vi "Boolean.vi"() -> ()   [LabVIEW 2020]
panel:
  out "0, 1":i16
  out "logical OR":bool
  out "logical AND":bool
  out "result":bool
  out ".not. (x .or. y)?":bool
  out "x .xor. y?":bool
  out "x .or. y?":bool
  out ".not. (x .and. y)?":bool
  out ".not. x?":bool
  in  "Boolean":bool
  out "x .and. y?":bool
  in  "x":bool
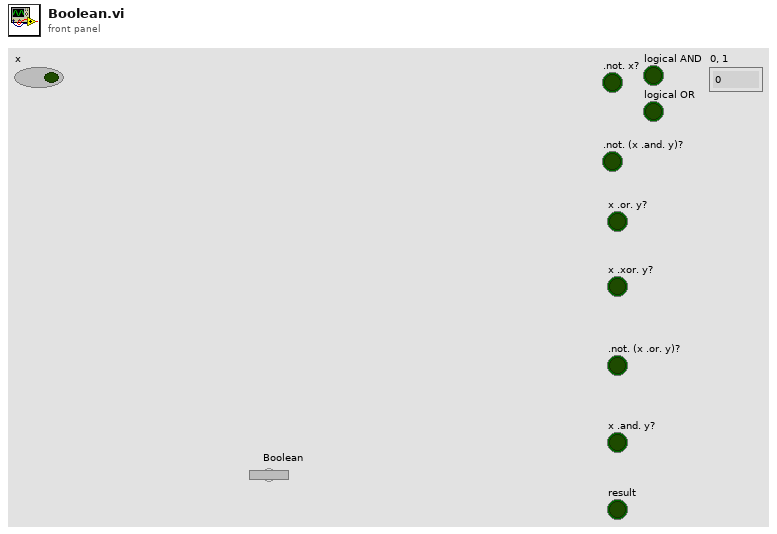
[diagram p1: front panel]
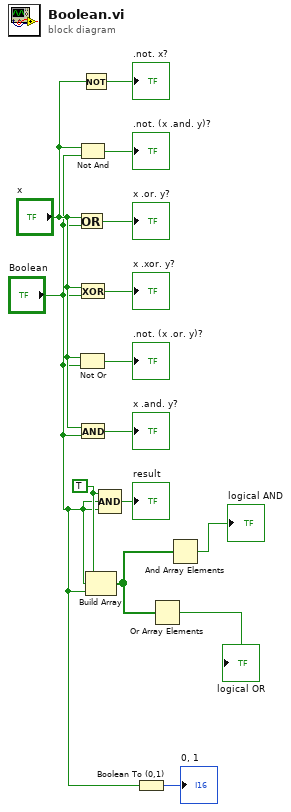
[diagram p0: block diagram]
diagram:
  w6 = TRUE
  n1 = Or(x="x", y="Boolean") -> (x .or. y?=→"x .or. y?":bool)
  n2 = Not Or(1:"Boolean", 2:"x") -> (0:→".not. (x .or. y)?":bool)
  n3 = Not And(1:"Boolean", 2:"x") -> (0:→".not. (x .and. y)?":bool)
  n4 = Exclusive Or(1:"Boolean", 2:"x") -> (0:→"x .xor. y?":bool)
  n5 = And(x="x", y="Boolean") -> (x .and. y?=→"x .and. y?":bool)
  n6 = Not(x="x") -> (.not. x?=→".not. x?":bool)
  n7 = Build Array(w6, "Boolean", "Boolean") -> (w5:bool[])
  n8 = Compound Arithmetic op=AND(w6, "Boolean", "Boolean") -> (→"result":bool)
  n9 = Boolean To (0,1)(Boolean="Boolean") -> (0, 1=→"0, 1":i16)
  n10 = Or Array Elements(Boolean array=w5) -> (logical OR=→"logical OR":bool)
  n11 = And Array Elements(Boolean array=w5) -> (logical AND=→"logical AND":bool)
